vi "Send Data to Arduino.vi"() -> ()   [LabVIEW 2013]
uses:
  Globals/Useful Values.vi
  Robot Global Data.vi
panel:
  out "error out":errorcluster
  out "Output String":string
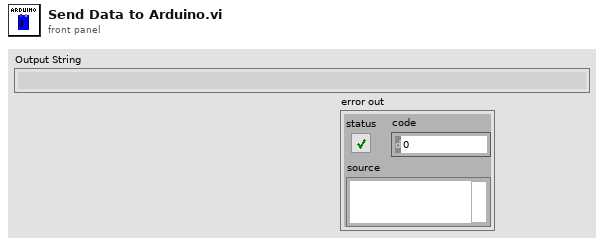
[diagram p1: front panel]
types:
  T1 = typedef "WPI_DriverStationRobotMode2.ctl" = enum16{"Autonomous Disabled", "Autonomous Enabled", "Teleop Disabled", "Teleop Enabled", "Timeout", "Finish", "Test Disabled", "Test Enabled"}
  T2 = typedef "WPI_DriverStationAllianceInfo.ctl" = enum16{"Red", "Blue", "Invalid"}
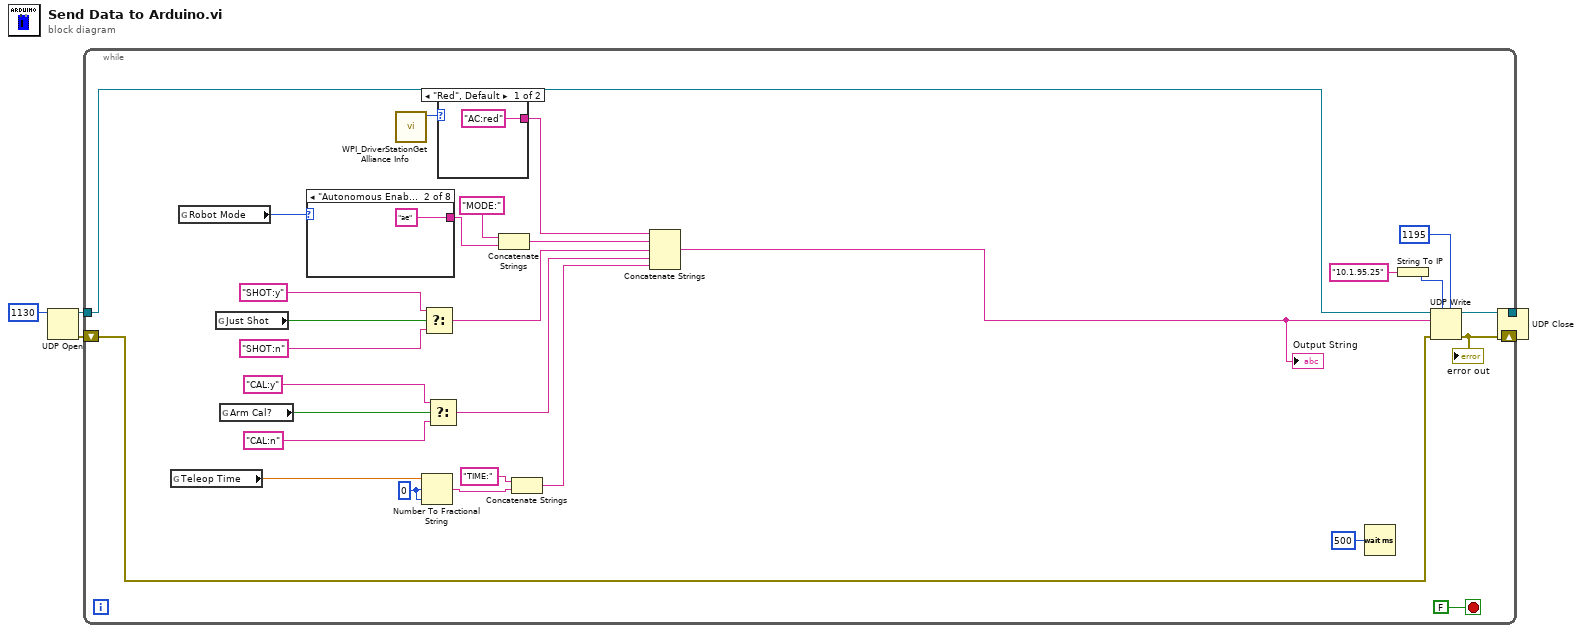
[diagram p0: block diagram]
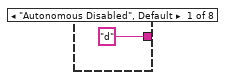
[diagram p2: hidden frame]
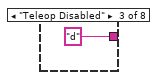
[diagram p3: hidden frame]
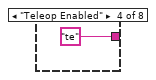
[diagram p4: hidden frame]
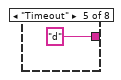
[diagram p5: hidden frame]
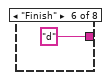
[diagram p6: hidden frame]
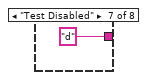
[diagram p7: hidden frame]
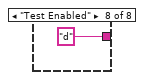
[diagram p8: hidden frame]
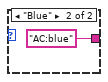
[diagram p9: hidden frame]
diagram:
  n1 = UDP Open(11:u16 1130 ("port")) -> (port=w4:refnum<k16>, 0:w3:errorcluster)  [unwired: 4 in, 1 out]
  n2 = while {
    tunnel: w4 -> [w23]
    shift-right: [w26] -> w2
    shift-left: w3 -> [w24]
    tunnel: [w25] -> w1
    stop <- FALSE stop-if-true
    w13 = i16 0 ("precision (6)")
    n3 = global read "Useful Values.vi" "Teleop Time"() -> (w14:dbl)
    n4 = global read "Robot Global Data.vi" "Robot Mode"() -> (w9:T1)
    n5 = global read "Useful Values.vi" "Just Shot"() -> (w30:bool)
    n6 = global read "Useful Values.vi" "Arm Cal?"() -> (w20:bool)
    n7 = case shown="\"Autonomous Enabled\"" w9 {
      tunnel: ["d" "ae" "d" "te" "d" "d" "d" "d"] -> w7
      frame "Autonomous Disabled", Default {
      }
      frame "Autonomous Enabled" {
      }
      frame "Teleop Disabled" {
      }
      frame "Teleop Enabled" {
      }
      frame "Timeout" {
      }
      frame "Finish" {
      }
      frame "Test Disabled" {
      }
      frame "Test Enabled" {
      }
    }
    n8 = call <vilib>:"WPI_DriverStationGet Alliance Info.vi"() -> ("Alliance"=w32:T2)  [unwired: 10 in, 1 out]
    n9 = Number To Fractional String(number=w14, width (-)=w13, precision (6)=w13) -> (F-format string=w12:string)  [unwired: 1 in]
    n10 = Select(t="SHOT:y", s=w30, f="SHOT:n") -> (s? t:f=w27:string)
    n11 = Select(t="CAL:y", s=w20, f="CAL:n") -> (s? t:f=w19:string)
    n12 = case shown="\"Red\", Default" w32 {
      tunnel: ["AC:red" "AC:blue"] -> w31
      frame "Red", Default {
      }
      frame "Blue" {
      }
    }
    n13 = Concatenate Strings("MODE:", w7) -> (w6:string)
    n14 = Concatenate Strings("TIME:" ("string"), w12) -> (w10:string)
    n15 = Concatenate Strings(w31, w6, w27, w19, w10) -> (w18:string)
    "Output String" <- w18
    n16 = Wait (ms)(milliseconds to wait=u32 500) -> ()  [unwired: 1 out]
    n17 = String To IP(1:"10.1.95.25" ("name")) -> (0:w16:u32)
    n18 = UDP Write(address=w16, port or service name=u16 1195, connection ID=w23, data in=w18, 8:w24) -> (error out=w26:errorcluster, 3:w25:refnum<k16>)  [unwired: 1 in]
    "error out" <- w26
  }
  n19 = UDP Close(connection ID=w1, 8:w2) -> ()  [unwired: 2 out]
